vi "HI.vi"(2 "error in (no error)":errorcluster, 3 "Image":T1, 4 "Matches (pixel)":T2(array[cluster]) {"Bounding Box"."y" format="%.2f"; "Bounding Box"."x" format="%.2f"; "Score" format="%.2f"; "Scale" format="%.2f"; "Angle" format="%.2f"; "Position"."y" format="%.2f"; "Position"."x" format="%.2f"}) -> (0 "error out":errorcluster, 1 "Image Out":T1)   [LabVIEW 2016]
uses:
  <vilib>/vision/Image Controls.llb/IMAQ Image.ctl
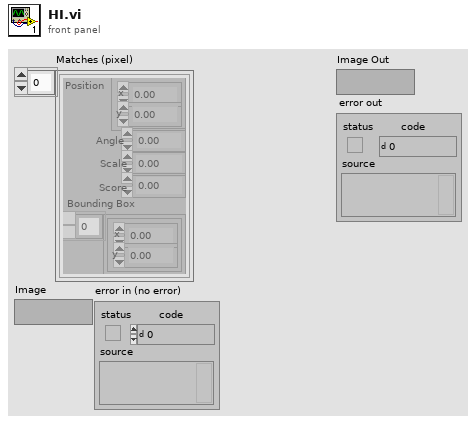
[diagram p1: front panel]
types:
  T1 = typedef "IMAQ Image.ctl" = refnum<image>
  T2 = cluster{"Position":cluster{"x":sgl, "y":sgl}, "Angle":sgl, "Scale":sgl, "Score":sgl, "Bounding Box":cluster{"x":sgl, "y":sgl}[]}[]
  T3 = cluster{"Position":cluster{"x":sgl, "y":sgl}, "Angle":sgl, "Scale":sgl, "Score":sgl, "Bounding Box":cluster{"x":sgl, "y":sgl}[]}
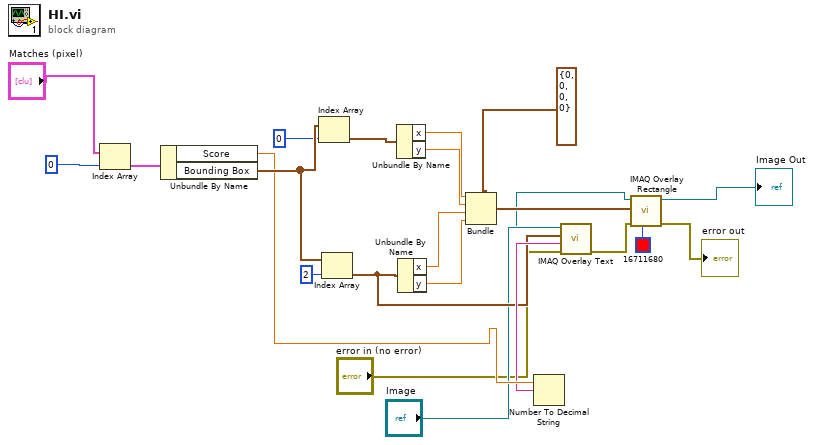
[diagram p0: block diagram]
diagram:
  n1 = Index Array(array="Matches (pixel)", index=0) -> (element=w21:T3)
  n2 = Unbundle By Name(w21) -> ("Score"=w10:sgl, "Bounding Box"=w20:cluster{"x":sgl, "y":sgl}[])
  n3 = Index Array(array=w20, index=0) -> (element=w17:cluster{"x":sgl, "y":sgl})
  n4 = Index Array(array=w20, index=2) -> (element=w6:cluster{"x":sgl, "y":sgl})
  n5 = Unbundle By Name(w17) -> ("x"=w15:sgl, "y"=w14:sgl)
  n6 = Unbundle By Name(w6) -> ("x"=w13:sgl, "y"=w12:sgl)
  n7 = Bundle(cluster=cluster{i32, i32, i32, i32} {0, 0, 0, 0} ("input cluster"), w15, w14, w13, w12) -> (w11:cluster{i32, i32, i32, i32})
  n8 = Number To Decimal String(number=w10) -> (decimal integer string=w8:string)  [unwired: 1 in]
  n9 = call "IMAQ Overlay Text"("error in (no error)"="error in (no error)", "String"=w8, "Origin"=w6, "Image"="Image") -> ("error out"=w2:errorcluster, "Image Out"=w4:T1)  [unwired: 6 in]
  n10 = call "IMAQ Overlay Rectangle"("Color"=u32 16711680, "error in (no error)"=w2, "Rectangle"=w11, "Image"=w4) -> ("error out"=→"error out":errorcluster, "Image Out"=→"Image Out":T1)  [unwired: 6 in]
